vi "create.vi"(0 "Object":refnum<class>, 2 "name":string, 5 "error in (no error)":errorcluster) -> (14 "HGF_Reference":refnum<class "HGF_Reference.lvclass">, 19 "error out":errorcluster)   [LabVIEW 2014, in "HGF_BaseClasses.lvlib" / "HGF_Reference.lvclass"]
doc: "Create a Reference object."
uses:
  HGF_Reference.lvclass
  HGF_Auxiliary/ErrorCode.ctl
  HGF_Auxiliary/Severity.ctl
  HGF_Reference.lvclass/HGF_Reference.ctl
  HGF_Auxiliary/HGF_Auxiliary.lvlib
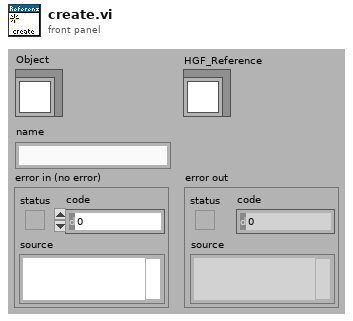
[diagram p1: front panel]
types:
  T1 = typedef "HGF_Auxiliary.lvlib/Severity.ctl" = enum16{"Info", "Warning", "Fault", "Error", "Fatal"}
  T2 = typedef "HGF_Auxiliary.lvlib/ErrorCode.ctl" = enum32{"No error", "Function not supported.", "This VI is for friends only.", "Reference object aready exisits.", "Parameter out of range.", "Not a rendezvous.", "Invalid notifier reference.", "Invalid queue reference.", "Self-Test not supported.", "Reset not supported.", "IDN query not supported.", "Error query not supported.", "Incorrect addressee.", "Object already exists.", "No class name specified", "Driver not supported", "Attribute is not writable"}
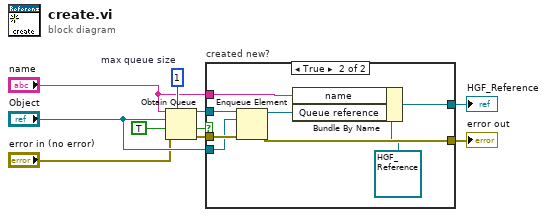
[diagram p0: block diagram]
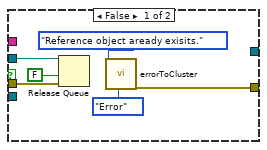
[diagram p2: hidden frame]
diagram:
  w10 = 1  # max queue size
  n1 = Obtain Queue(max queue size (-1, unlimited)=w10, name (unnamed)="name", element data type="Object", create if not found? (T)=TRUE, error in (no error)="error in (no error)") -> (queue out=w8:refnum<queue>, created new?=w6:bool, error out=w9:errorcluster)
  n2 = case "created new?" shown="True" w6 {
    tunnel: w9 -> [w15 w23]
    tunnel: w8 -> [w16 w22]
    tunnel: "Object" -> [_ w21]
    tunnel: [_ w20] -> w3
    tunnel: [w13 w19] -> w2
    tunnel: "name" -> [_ w18]
    frame False {
      n3 = Release Queue(queue=w16, force destroy? (F)=FALSE, error in (no error)=w15) -> ()  [unwired: 3 out]
      n4 = call "errorToCluster.vi"("error code"=ErrorCode."Reference object aready exisits.", "severity (Error)"=Severity."Error") -> ("error out"=w13:errorcluster)  [unwired: 3 in, 14 out]
    }
    frame True {
      n5 = Enqueue Element(queue=w22, element=w21, error in (no error)=w23) -> (queue out=w24:refnum<queue>, error out=w19:errorcluster)  [unwired: 2 out]
      n6 = Bundle By Name(cluster=refnum<class "HGF_Reference.lvclass"> refnum ("HGF_Reference.lvclass"), "name"=w18, "Queue reference"=w24) -> (w20:refnum<class "HGF_Reference.lvclass">)
    }
  }
  "HGF_Reference" <- w3
  "error out" <- w2
